vi "ReadRxStats.vi"(8 "error in (no error)":errorcluster, 11 "reference in":refnum<class "WebSocket.lvclass">) -> (0 "error out":errorcluster, 2 "Stats":T1, 3 "reference out":refnum<class "WebSocket.lvclass">)   [LabVIEW 2023, in "WebSocket.lvclass"]
uses:
  WebSocket.lvclass
  Stats.ctl
  WebSocket Stats VIG Mode.ctl
  WebSocket Stats.ctl
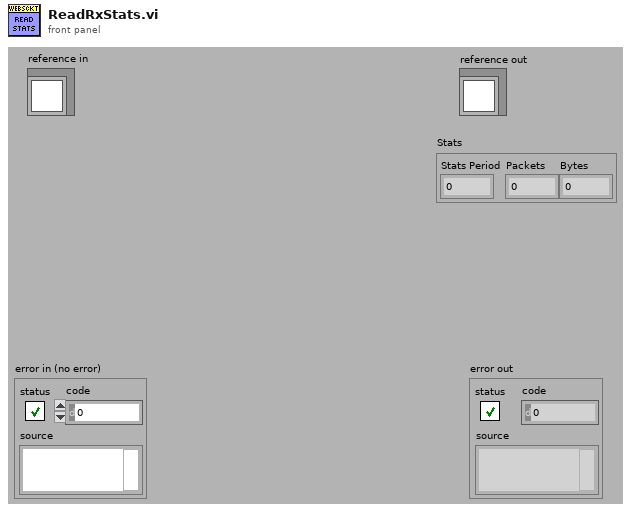
[diagram p1: front panel]
types:
  T1 = typedef "WebSocket.lvclass/Stats.ctl" = cluster{"Stats Period":dbl, "Packets":u64, "Bytes":u64}
  T2 = typedef "WebSocket Stats.ctl" = cluster{"T0":timestamp, "Tlast":timestamp, "Bytes":i32, "Packets":i32}
  T3 = typedef "WebSocket Stats VIG Mode.ctl" = enum16{"Init", "Set", "Update", "Get All"}
  T4 = typedef "WebSocket.lvclass/ObjectAttributes.ctl" = cluster{"Socket":refnum<k5>, "Thread":refnum<vi>, "From Socket":refnum<queue>, "To Socket":refnum<queue>, "Rx Stats in Progress":variant, "Rx Stats":variant, "Tx Stats in Progress":variant, "Tx Stats":variant}
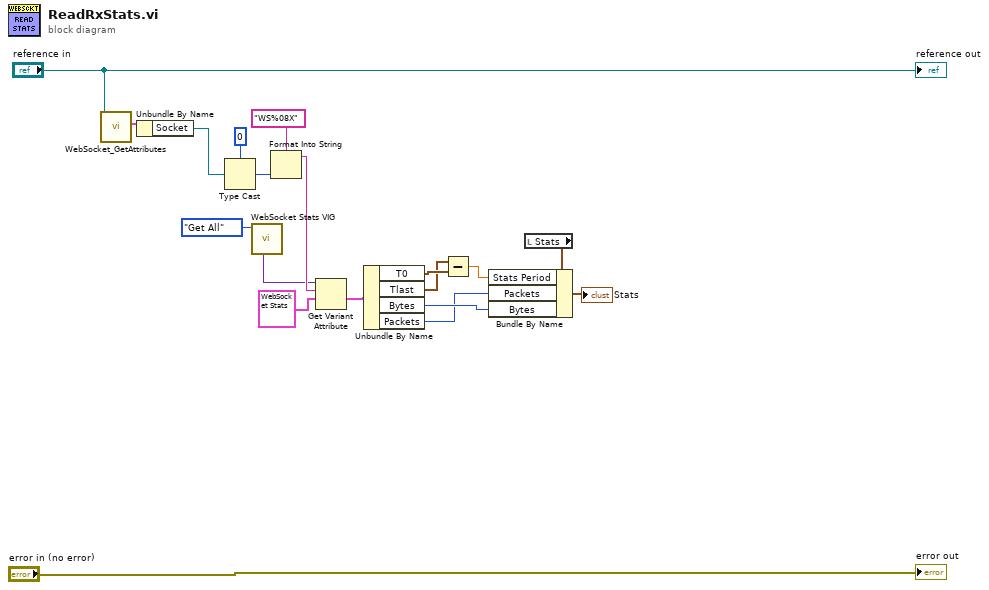
[diagram p0: block diagram]
diagram:
  n1 = call "WebSocket_GetAttributes.vi"("reference in"="reference in") -> ("Data"=w12:T4)  [unwired: 7 in, 3 out]
  n2 = Unbundle By Name(w12) -> ("Socket"=w11:refnum<k5>)
  n3 = Type Cast(type=0, x=w11) -> (*(type *) &x=w14:i32)
  n4 = call "WebSocket Stats VIG.vi"("mode"=WebSocket_Stats_VIG_Mode."Get All") -> ("RX Stats"=w4:variant)  [unwired: 8 in, 2 out]
  n5 = Format Into String(format string="WS%08X", w14) -> (resulting string=w10:string)  [unwired: 2 in, 1 out]
  n6 = Get Variant Attribute(Variant=w4, name=w10, default value (empty Variant)=T2 {"T0"=timestamp(0 s since 1904-01-01), "Tlast"=timestamp(0 s since 1904-01-01), "Bytes"=0, "Packets"=0} ("Socket Stats")) -> (value=w8:T2)  [unwired: 1 in, 3 out]
  n7 = Unbundle By Name(w8) -> ("T0"=w7:timestamp, "Tlast"=w6:timestamp, "Bytes"=w3:i32, "Packets"=w2:i32)
  n8 = Subtract(x=w6, y=w7) -> (x-y=w1:dbl)
  n9 = local read "Stats"() -> (w19:T1)
  n10 = Bundle By Name(cluster=w19, "Stats Period"=w1, "Packets"=w2, "Bytes"=w3) -> (→"Stats":T1)
  "error out" <- "error in (no error)"
  "reference out" <- "reference in"
